vi "run.update_add_label.vi"(8 "error in":errorcluster, 11 "RunUpdateStaging in":refnum<class "RunUpdateStaging.lvclass">) -> (0 "error out":errorcluster, 3 "RunUpdateStaging out":refnum<class "RunUpdateStaging.lvclass">)   [LabVIEW 2020, in "RunUpdateStaging.lvclass"]
doc: "Adds a label to the staged update, replacing the run's entire label set with the accumulated labels when applied."
uses:
  RunUpdateStaging.lvclass
  RunUpdateStaging.lvclass/RunUpdateStaging.ctl
  client.lvlib
panel:
  in  "label":string
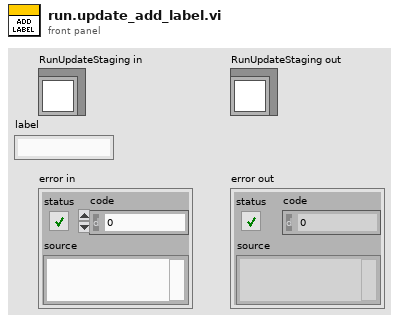
[diagram p1: front panel]
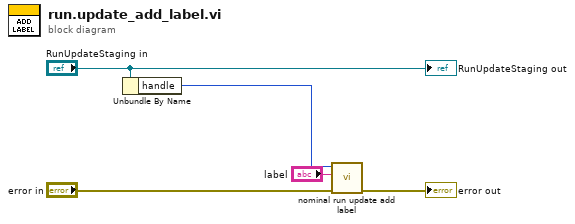
[diagram p0: block diagram]
diagram:
  n1 = Unbundle By Name("RunUpdateStaging in") -> ("handle"=w3:i32)
  n2 = call "nominal run update add label.vi"("error in (no error)"="error in", "label"="label", "staging"=w3) -> ("error out"=→"error out":errorcluster)  [unwired: 7 in, 1 out]
  "RunUpdateStaging out" <- "RunUpdateStaging in"
